vi "EnQueue-N.vi"(8 "error in (no error)":errorcluster, 10 "Array Of States":string[](array[string]), 11 "queue ref":refnum<queue>) -> (0 "error out":errorcluster, 3 "queue out":refnum<queue>)   [LabVIEW 2022 SP3]
doc: "Use this template to build a VI to use as a subVI."
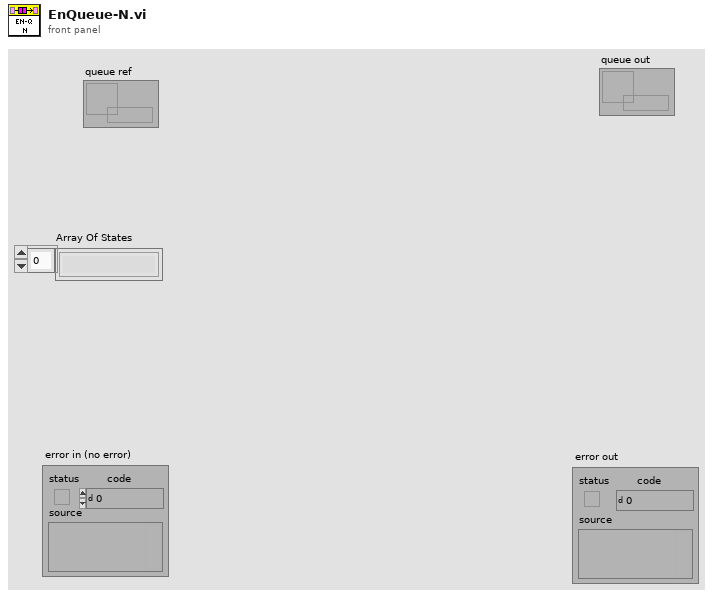
[diagram p1: front panel]
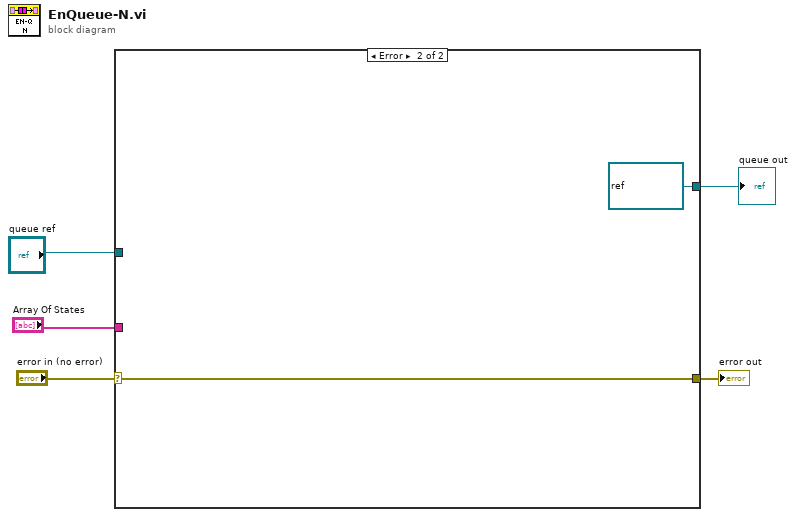
[diagram p0: block diagram]
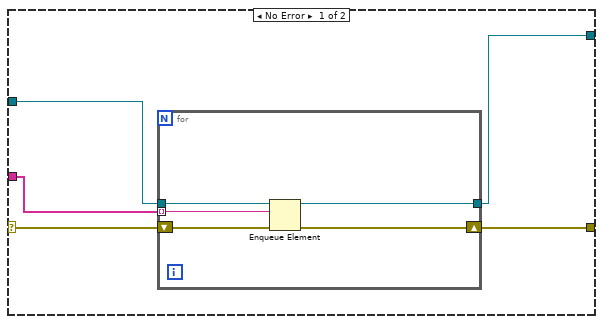
[diagram p2: hidden frame]
diagram:
  n1 = case shown="Error" "error in (no error)" {
    selector: "error in (no error)" -> [w10 w17]
    tunnel: [w9 w17] -> w4
    tunnel: "queue ref" -> [w8 _]
    tunnel: "Array Of States" -> [w7 _]
    tunnel: [w6 refnum<queue> refnum ("queue ref")] -> w1
    frame No Error {
      n2 = for {
        tunnel: w8 -> [w13]
        shift-right: [w14] -> w9
        shift-left: w10 -> [w15]
        tunnel: w7 -> [w12] mode=indexing
        tunnel: [w11] -> w6
        n3 = Enqueue Element(queue=w13, element=w12, error in (no error)=w15) -> (queue out=w11:refnum<queue>, error out=w14:errorcluster)  [unwired: 1 in, 1 out]
      }
    }
    frame Error {
    }
  }
  "error out" <- w4
  "queue out" <- w1
